vi "Read_only_Manipulator.vi"(5 "waiting time (ms)":u32, 6 "Print?":bool, 7 "Motor":u16(ring) items=["none", "1", "2", "3", "4", "all"], 8 "error in (no error)":errorcluster, 9 "Value":string, 10 "Command":T1=enum."Move Relative (MR)", 11 "VISA resource name":refnum<visa-resource-name>) -> (0 "error out":errorcluster={"status"=FALSE, "code"=1073676294, "source"="VISA Read in write_read.vi"}, 1 "Transmitted String":string, 3 "VISA ressource out":refnum<visa-resource-name>, 4 "Motor Moving":string)   [LabVIEW 2018]
uses:
  MCode_LV_86/Set Parameter.ctl
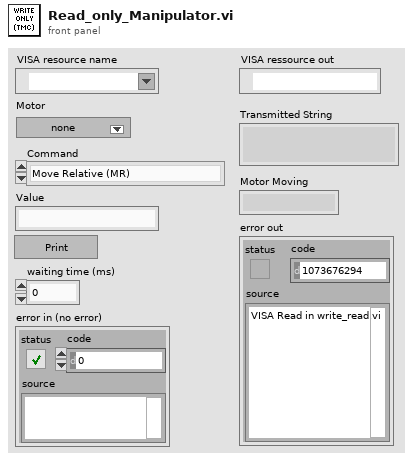
[diagram p1: front panel]
types:
  T1 = typedef "Set Parameter.ctl" = enum16{"Acceleration (A)", "Baud Rate (BD)", "Counter 1 (C1)", "Counter 2 (C2)", "Control C Software Reset (CE)", "Check Sum Enable (CK)", "Clock Mode (CM)", "Clock Mode Ratio (CR)", "Clock Mode Out Step Width (CW)", "Deceleration (D)", "Digital Filtering, Input 1 (D1)", "Digital Filtering, Input 2 (D2)", "Digital Filtering, Input 3 (D3)", "Digital Filtering, Input 4 (D4)", "Digital Filtering, Input 5 (D5)", "Digital Filtering, Input 9 (D9)", "Digital Filtering, Input 10 (D10)", "Digital Filtering, Input 11 (D11)", "Digital Filtering, Input 12 (D12)", "Deadband (DB)", "Decrement Variable (DC)", "Enable/Disable Drive (DE)", "Device Name (DN)", "End Program Execution (E)", "Encoder Function Enable (EE)", "Error Flag (EF)", "Encoder Lines (EL)", "Echo Mode (EM)", "Error Value (ER)", "Escape (ES)", "Execute Program at Address (EX)", "Firmware Version (VR)", "Hold (H)", "Hold Current (HC)", "Hold Current Delay Time (HI)", "Home to Encoder Index (HM)", "Home to Home Switch (HT)", "Increment Variable (IC)", "Initialize Parameters to NVM (IP)", "Input into Variable (IV)", "Jog Enable (JE)", "Limit Stop Mode (LM)", "Move Absolute (MA)", "Move Relative (MR)", "MicroStepping Select (MS)", "Motor Settling Delay Time (MT)", "Moving [Flag] (MV)", "Output 1 (O1)", "Output 2 (O2)", "Output 3 (O3)", "Output 4 (O4)", "Output 9 (O9)", "Output 10 (O10)", "Output 11 (O11)", "Output 12 (O12)", "Output High Byte (9-12) (OH)", "Output Low Byte (1-4) (OL)", "Output Total (1-4 and 9-12) (OT)", "Position (P)", "Position Maintenance (PM)", "Party Mode (PY)", "Register 1 (R1)", "Register 2 (R2)", "Register 3 (R3)", "Register 4 (R4)", "Reset Error(\\03)", "Run Current (RC)", "Stall Factor (SF)", "Slew (SL)", "Stall Mode Set (SM)", "Upgrade Firmware (UG)", "Velocity Initial (VI)", "Velocity Maximum (VM)", "Current1 (I1)", "Current2 (I2)", "Current3 (I3)", "Current4 (I4)", "Current5 (I5)", "Current6 (I6)", "Save (S)"}
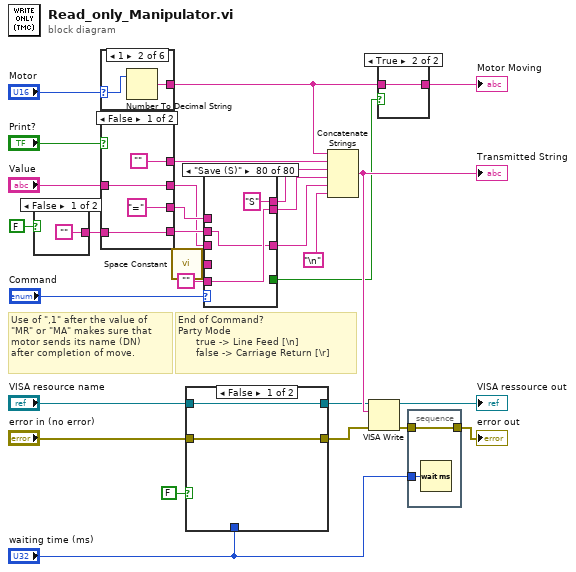
[diagram p0: block diagram]
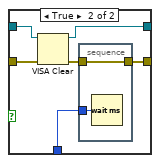
[diagram p2: hidden frame]
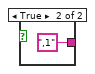
[diagram p3: hidden frame]
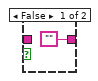
[diagram p4: hidden frame]
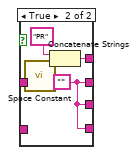
[diagram p5: hidden frame]
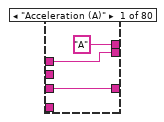
[diagram p6: hidden frame]
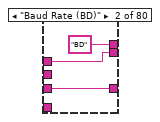
[diagram p7: hidden frame]
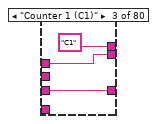
[diagram p8: hidden frame]
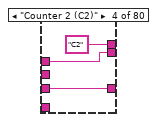
[diagram p9: hidden frame]
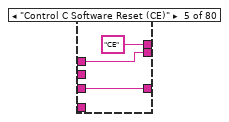
[diagram p10: hidden frame]
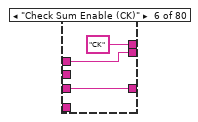
[diagram p11: hidden frame]
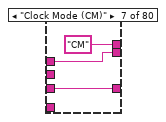
[diagram p12: hidden frame]
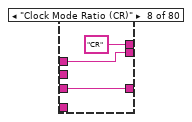
[diagram p13: hidden frame]
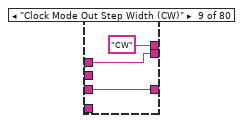
[diagram p14: hidden frame]
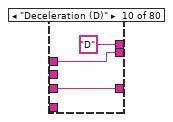
[diagram p15: hidden frame]
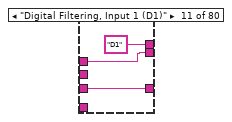
[diagram p16: hidden frame]
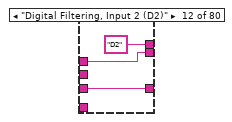
[diagram p17: hidden frame]
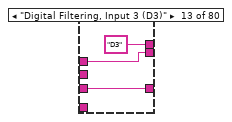
[diagram p18: hidden frame]
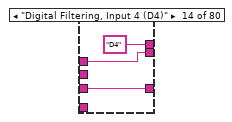
[diagram p19: hidden frame]
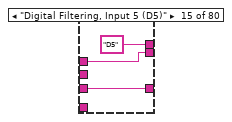
[diagram p20: hidden frame]
diagram:
  # "Use of \",1\" after the value of\n\"MR\" or \"MA\" makes sure that\nmotor sends its name (DN) \nafter completion of move."
  # "End of Command?\nParty Mode \n      true -> Line Feed [\\n]\n      false -> Carriage Return [\\r]"
  n1 = case shown="False" FALSE {
    tunnel: ["" ",1"] -> w7
    frame False {
    }
    frame True {
    }
  }
  n2 = case shown="1" "Motor" {
    selector: "Motor" -> [_ w33 w35 w37 w39 _]
    tunnel: ["" w34 w36 w38 w40 "*"] -> w10
    frame 0, Default {
    }
    frame 1 {
      n3 = Number To Decimal String(number=w33) -> (decimal integer string=w34:string)  [unwired: 1 in]
    }
    frame 2 {
      n4 = Number To Decimal String(number=w35) -> (decimal integer string=w36:string)  [unwired: 1 in]
    }
    frame 3 {
      n5 = Number To Decimal String(number=w37) -> (decimal integer string=w38:string)  [unwired: 1 in]
    }
    frame 4 {
      n6 = Number To Decimal String(number=w39) -> (decimal integer string=w40:string)  [unwired: 1 in]
    }
    frame 5 {
    }
  }
  n7 = case shown="False" "Print?" {
    tunnel: ["" w48] -> w25
    tunnel: "Value" -> [w45 _]
    tunnel: [w45 w46] -> w17
    tunnel: ["=" w46] -> w19
    tunnel: [w42 w46] -> w18
    tunnel: w7 -> [w42 _]
    frame False {
    }
    frame True {
      w46 = ""
      n8 = call <vilib>:"Space Constant.vi"() -> ("String"=w49:string)
      n9 = Concatenate Strings("PR" ("string"), w49) -> (w48:string)
    }
  }
  n10 = call <vilib>:"Space Constant.vi"() -> ("String"=w24:string)
  n11 = case shown="False" FALSE {
    tunnel: "waiting time (ms)" -> [_ w57]
    tunnel: "error in (no error)" -> [w50 w56]
    tunnel: "VISA resource name" -> [w51 w54]
    tunnel: [w51 w53] -> w3
    tunnel: [w50 w52] -> w2
    frame False {
    }
    frame True {
      n12 = VISA Clear(VISA resource name=w54, error in (no error)=w56) -> (VISA resource name out=w53:refnum<visa-resource-name>, error out=w55:errorcluster)
      n13 = stacked-sequence {
        tunnel: w55 -> [w59]
        tunnel: [w59] -> w52
        tunnel: w57 -> [w58]
        frame #0 {
          n14 = Wait (ms)(milliseconds to wait=w58) -> ()  [unwired: 1 out]
        }
      }
    }
  }
  n15 = case shown="\"Save (S)\"" "Command" {
    tunnel: ["A" ("string") "BD" ("string") "C1" ("string") "C2" ("string") "CE" ("string") "CK" ("string") "CM" ("string") "CR" ("string") "CW" ("string") "D" ("string") "D1" ("string") "D2" ("string") "D3" ("string") "D4" ("string") "D5" ("string") "D9" ("string") "D10" ("string") "D11" ("string") "D12" ("string") "DB" ("string") "DC" ("string") "DE" ("string") "DN" ("string") "E" ("string") "EE" ("string") "EF" ("string") "EM" ("string") "ER" ("string") "ES" ("string") "EX" ("string") "VR" ("string") "H" ("string") "HC" ("string") "HI" ("string") "HM" ("string") "HT" ("string") "IC" ("string") "IP" ("string") "IV" ("string") "JE" ("string") "LM" ("string") "MA" ("string") "MR" ("string") "MS" ("string") "MT" ("string") "O1" ("string") "O2" ("string") "O3" ("string") "O4" ("string") "O9" ("string") "O10" ("string") "O11" ("string") "O12" ("string") "OH" ("string") "OL" ("string") "OT" ("string") "P" ("string") "PM" ("string") "PY" ("string") "R1" ("string") "R2" ("string") "R3" ("string") "R4" ("string") "RC" ("string") "SF" ("string") "SL" ("string") "SM" ("string") "UG" ("string") "VI" ("string") "VM" ("string") "EL" ("string") "\u0003" "MV" ("string") "I1" ("string") "I2" ("string") "I3" ("string") "I4" ("string") "I5" ("string") "I6" ("string") "S" ("string")] -> w27
    tunnel: w19 -> [w61 w64 w67 w70 w73 w76 w79 w82 w85 w88 w91 w94 w97 w100 w103 w106 w109 w112 w115 w118 w121 w124 w127 _ w133 w137 w139 w142 w145 w148 _ _ w157 w160 w163 w166 w169 w172 w175 w178 w181 _ _ w196 w199 w202 w205 w208 w211 w214 w217 w220 w223 w226 w229 w232 w236 w238 w241 w244 w247 w250 w253 w256 w259 w262 w265 w268 w271 w274 w277 _ _ w286 w289 w291 w294 w297 w300 _]
    tunnel: w24 -> [_ _ _ _ _ _ _ _ _ _ _ _ _ _ _ _ _ _ _ _ _ _ _ _ _ _ _ _ _ _ _ _ _ _ _ _ _ _ _ _ _ w188 w194 _ _ _ _ _ _ _ _ _ _ _ _ _ _ _ _ _ _ _ _ _ _ _ _ _ _ _ _ _ _ _ _ _ _ _ _ _]
    tunnel: [w61 w64 w67 w70 w73 w76 w79 w82 w85 w88 w91 w94 w97 w100 w103 w106 w109 w112 w115 w118 w121 w124 w127 w130 w133 w137 w139 w142 w145 w148 w152 w154 w157 w160 w163 w166 w169 w172 w175 w178 w181 w188 w194 w196 w199 w202 w205 w208 w211 w214 w217 w220 w223 w226 w229 w232 w236 w238 w241 w244 w247 w250 w253 w256 w259 w262 w265 w268 w271 w274 w277 w281 w283 w286 w289 w291 w294 w297 w300 w304] -> w22
    tunnel: "" -> [_ _ _ _ _ _ _ _ _ _ _ _ _ _ _ _ _ _ _ _ _ _ _ w130 _ _ _ _ _ _ w152 w154 _ _ _ _ _ _ _ _ _ _ _ _ _ _ _ _ _ _ _ _ _ _ _ _ _ _ _ _ _ _ _ _ _ _ _ _ _ _ _ w281 w283 _ _ _ _ _ _ w304]
    tunnel: w18 -> [_ _ _ _ _ _ _ _ _ _ _ _ _ _ _ _ _ _ _ _ _ _ _ _ _ _ _ _ _ _ _ _ _ _ _ _ _ _ _ _ _ w185 w190 _ _ _ _ _ _ _ _ _ _ _ _ _ _ _ _ _ _ _ _ _ _ _ _ _ _ _ _ _ _ _ _ _ _ _ _ w303]
    tunnel: w17 -> [w60 w63 w66 w69 w72 w75 w78 w81 w84 w87 w90 w93 w96 w99 w102 w105 w108 w111 w114 w117 w120 w123 w126 w129 w132 w135 w138 w141 w144 w147 w150 w153 w156 w159 w162 w165 w168 w171 w174 w177 w180 w187 w191 w195 w198 w201 w204 w207 w210 w213 w216 w219 w222 w225 w228 w231 w234 w237 w240 w243 w246 w249 w252 w255 w258 w261 w264 w267 w270 w273 w276 w279 w284 w285 w288 w293 w296 w299 w302 _]
    tunnel: [w60 w63 w66 w69 w72 w75 w78 w81 w84 w87 w90 w93 w96 w99 w102 w105 w108 w111 w114 w117 w120 w123 w126 w129 w132 w135 w138 w141 w144 w147 w150 w153 w156 w159 w162 w165 w168 w171 w174 w177 w180 w184 w192 w195 w198 w201 w204 w207 w210 w213 w216 w219 w222 w225 w228 w231 w234 w237 w240 w243 w246 w249 w252 w255 w258 w261 w264 w267 w270 w273 w276 w279 w284 w285 w288 w293 w296 w299 w302 w303] -> w16
    tunnel: [_ _ _ _ _ _ _ _ _ _ _ _ _ _ _ _ _ _ _ _ _ _ _ _ _ _ _ _ _ _ _ _ _ _ _ _ _ _ _ _ _ TRUE TRUE _ _ _ _ _ _ _ _ _ _ _ _ _ _ _ _ _ _ _ _ _ _ _ _ _ _ _ _ _ _ _ _ _ _ _ _ _] -> w11
    frame "Acceleration (A)" {
    }
    frame "Baud Rate (BD)" {
    }
    frame "Counter 1 (C1)" {
    }
    frame "Counter 2 (C2)" {
    }
    frame "Control C Software Reset (CE)" {
    }
    frame "Check Sum Enable (CK)" {
    }
    frame "Clock Mode (CM)" {
    }
    frame "Clock Mode Ratio (CR)" {
    }
    frame "Clock Mode Out Step Width (CW)" {
    }
    frame "Deceleration (D)" {
    }
    frame "Digital Filtering, Input 1 (D1)" {
    }
    frame "Digital Filtering, Input 2 (D2)" {
    }
    frame "Digital Filtering, Input 3 (D3)" {
    }
    frame "Digital Filtering, Input 4 (D4)" {
    }
    frame "Digital Filtering, Input 5 (D5)" {
    }
    frame "Digital Filtering, Input 9 (D9)" {
    }
    frame "Digital Filtering, Input 10 (D10)" {
    }
    frame "Digital Filtering, Input 11 (D11)" {
    }
    frame "Digital Filtering, Input 12 (D12)" {
    }
    frame "Deadband (DB)" {
    }
    frame "Decrement Variable (DC)" {
    }
    frame "Enable/Disable Drive (DE)" {
    }
    frame "Device Name (DN)" {
    }
    frame "End Program Execution (E)" {
    }
    frame "Encoder Function Enable (EE)" {
    }
    frame "Error Flag (EF)" {
    }
    frame "Echo Mode (EM)" {
    }
    frame "Error Value (ER)" {
    }
    frame "Escape (ES)" {
    }
    frame "Execute Program at Address (EX)" {
    }
    frame "Firmware Version (VR)" {
    }
    frame "Hold (H)" {
    }
    frame "Hold Current (HC)" {
    }
    frame "Hold Current Delay Time (HI)" {
    }
    frame "Home to Encoder Index (HM)" {
    }
    frame "Home to Home Switch (HT)" {
    }
    frame "Increment Variable (IC)" {
    }
    frame "Initialize Parameters to NVM (IP)" {
    }
    frame "Input into Variable (IV)" {
    }
    frame "Jog Enable (JE)" {
    }
    frame "Limit Stop Mode (LM)" {
    }
    frame "Move Absolute (MA)" {
      n16 = Concatenate Strings(w187, w185) -> (w184:string)
    }
    frame "Move Relative (MR)" {
      n17 = Concatenate Strings(w191, w190) -> (w192:string)
    }
    frame "MicroStepping Select (MS)" {
    }
    frame "Motor Settling Delay Time (MT)" {
    }
    frame "Output 1 (O1)" {
    }
    frame "Output 2 (O2)" {
    }
    frame "Output 3 (O3)" {
    }
    frame "Output 4 (O4)" {
    }
    frame "Output 9 (O9)" {
    }
    frame "Output 10 (O10)" {
    }
    frame "Output 11 (O11)" {
    }
    frame "Output 12 (O12)" {
    }
    frame "Output High Byte (9-12) (OH)" {
    }
    frame "Output Low Byte (1-4) (OL)" {
    }
    frame "Output Total (1-4 and 9-12) (OT)" {
    }
    frame "Position (P)" {
    }
    frame "Position Maintenance (PM)" {
    }
    frame "Party Mode (PY)" {
    }
    frame "Register 1 (R1)" {
    }
    frame "Register 2 (R2)" {
    }
    frame "Register 3 (R3)" {
    }
    frame "Register 4 (R4)" {
    }
    frame "Run Current (RC)" {
    }
    frame "Stall Factor (SF)" {
    }
    frame "Slew (SL)" {
    }
    frame "Stall Mode Set (SM)" {
    }
    frame "Upgrade Firmware (UG)" {
    }
    frame "Velocity Initial (VI)" {
    }
    frame "Velocity Maximum (VM)" {
    }
    frame "Encoder Lines (EL)" {
    }
    frame "Reset Error(\\03)" {
    }
    frame "Moving [Flag] (MV)" {
    }
    frame "Current1 (I1)" {
    }
    frame "Current2 (I2)" {
    }
    frame "Current3 (I3)" {
    }
    frame "Current4 (I4)" {
    }
    frame "Current5 (I5)" {
    }
    frame "Current6 (I6)" {
    }
    frame "Save (S)" {
    }
  }
  n18 = Concatenate Strings(w10, w25, w27, w22, w16, "\n") -> (w20:string)
  "Transmitted String" <- w20
  n19 = VISA Write(VISA resource name=w3, write buffer=w20, error in (no error)=w2) -> (VISA resource name out=→"VISA ressource out":refnum<visa-resource-name>, error out=w14:errorcluster)  [unwired: 1 out]
  n20 = case shown="True" w11 {
    tunnel: w10 -> [_ w307]
    tunnel: ["" w307] -> w9
    frame False {
    }
    frame True {
    }
  }
  "Motor Moving" <- w9
  n21 = stacked-sequence {
    tunnel: w14 -> [w309]
    tunnel: [w309] -> w13
    tunnel: "waiting time (ms)" -> [w308]
    frame #0 {
      n22 = Wait (ms)(milliseconds to wait=w308) -> ()  [unwired: 1 out]
    }
  }
  "error out" <- w13
